vi "Configure Arming (Time).vi"(0 "VISA resource name":refnum<visa-resource-name>, 1 "Measurement (0:Frequency)":i32(ring) items=["Frequency", "Frequency Ratio", "Period", "Totalize", "Phase", "Edge Rise Time", "Edge Fall Time", "Positive Pulse Width", "Negative Pulse Width", "Duty Cycle", "Time Interval", "Volt Maximum", "Volt Minimum"], 5 "Arm Time (0.1s)":dbl=0.1 format="%^#.5g", 11 "error in (no error)":errorcluster) -> (4 "VISA resource name out":refnum<visa-resource-name>, 15 "error out":errorcluster)   [LabVIEW 2020, in "Counter.lvlib" / "PICOTEST U62XXA series.lvlib"]
doc: "Configures the parameters for Time Arming.This VI should be called after the Configure Measurement VI.\n\n<B>Note:</B>\n\n<B>Only</B> Frequency, Frequency Ratio, Period and Totalize have Time Arming capabilities."
uses:
  PICOTEST U62XXA series.lvlib
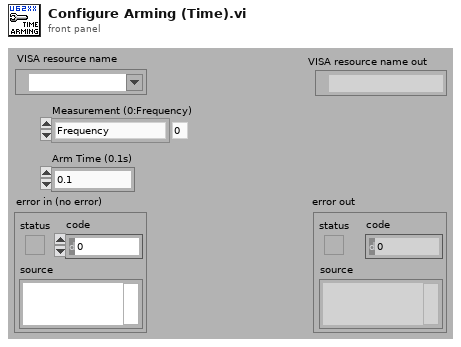
[diagram p1: front panel]
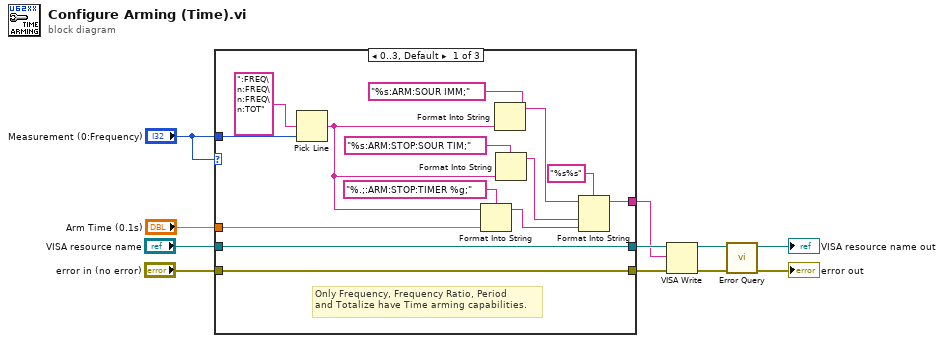
[diagram p0: block diagram]
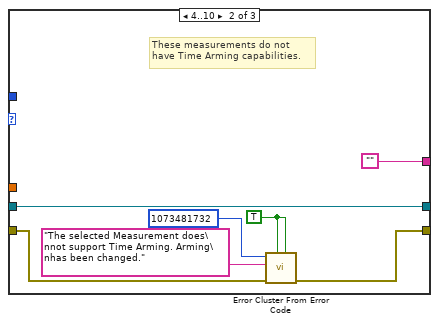
[diagram p2: hidden frame]
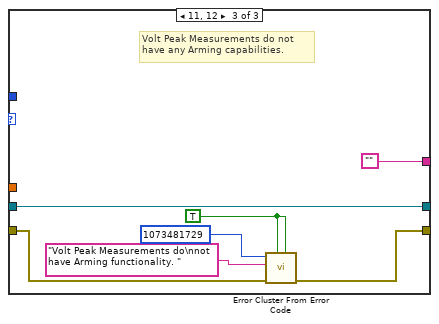
[diagram p3: hidden frame]
diagram:
  n1 = case shown="0..3, Default" "Measurement (0:Frequency)" {
    tunnel: [w15 "" ""] -> w1
    tunnel: "Measurement (0:Frequency)" -> [w23 _ _]
    tunnel: "Arm Time (0.1s)" -> [w22 _ _]
    tunnel: "VISA resource name" -> [w21 w30 w37]
    tunnel: [w21 w30 w37] -> w4
    tunnel: "error in (no error)" -> [w20 w29 w36]
    tunnel: [w20 w28 w35] -> w2
    frame 0..3, Default {
      # "Only Frequency, Frequency Ratio, Period\nand Totalize have Time arming capabilities."
      n2 = Pick Line(multi-line string=":FREQ\n:FREQ\n:FREQ\n:TOT", line index=w23) -> (output string=w17:string)  [unwired: 1 in]
      n3 = Format Into String(format string="%.;:ARM:STOP:TIMER %g;", initial string=w17, w22) -> (resulting string=w12:string)  [unwired: 1 in, 1 out]
      n4 = Format Into String(format string="%s:ARM:SOUR IMM;", w17) -> (resulting string=w16:string)  [unwired: 2 in, 1 out]
      n5 = Format Into String(format string="%s:ARM:STOP:SOUR TIM;", w17) -> (resulting string=w13:string)  [unwired: 2 in, 1 out]
      n6 = Format Into String(format string="%s%s", initial string=w16, w13, w12) -> (resulting string=w15:string)  [unwired: 1 in, 1 out]
    }
    frame 4..10 {
      w31 = TRUE ("is warning? (False)")
      # "These measurements do not\nhave Time Arming capabilities."
      n7 = call <vilib>:"Error Cluster From Error Code.vi"("is warning? (False)"=w31, "show call chain? (False)"=w31, "error in (no error)"=w29, "error message (\"\")"="The selected Measurement does\nnot support Time Arming. Arming\nhas been changed." ("error message (\"\")"), "error code (0)"=1073481732 ("Code")) -> ("error out"=w28:errorcluster)  [unwired: 4 in]
    }
    frame 11, 12 {
      w38 = TRUE ("is warning? (False)")
      # "Volt Peak Measurements do not \nhave any Arming capabilities."
      n8 = call <vilib>:"Error Cluster From Error Code.vi"("is warning? (False)"=w38, "show call chain? (False)"=w38, "error in (no error)"=w36, "error message (\"\")"="Volt Peak Measurements do\nnot have Arming functionality. " ("error message (\"\")"), "error code (0)"=1073481729 ("Code")) -> ("error out"=w35:errorcluster)  [unwired: 4 in]
    }
  }
  n9 = VISA Write(VISA resource name=w4, write buffer=w1, error in (no error)=w2) -> (VISA resource name out=w11:refnum<visa-resource-name>, error out=w10:errorcluster)  [unwired: 1 out]
  n10 = call "Error Query.vi"("error in (no error)"=w10, "VISA resource name"=w11) -> ("error out"=→"error out":errorcluster, "VISA resource name out"=→"VISA resource name out":refnum<visa-resource-name>)  [unwired: 6 in, 2 out]
